vi "Start.vi"(1 "Engine":refnum<k7>, 2 "Context":refnum<k7>) -> (0 "Error Out":errorcluster)   [LabVIEW 2021, in "Seq Edit Quick Drop.lvlib"]
uses:
  Seq Edit Quick Drop.lvlib
  Command.ctl
  Data.ctl
  Register Item.ctl
  Message.ctl
  Event Response.ctl
  Connection Type.ctl
  Combine Key with Modifiers.vi
  Get Modifier from Key Event.vi
  Get Modifier.vi
  Scan Codes Mapping.vi
  <vilib>/Utility/error.llb/Trim Whitespace.vi
  Settings.vi
  <vilib>/Utility/SystemLogging/NI_SystemLogging.lvlib
  Resources/Tool Menu Utility.lvlibp/Tools/Tools.lvclass
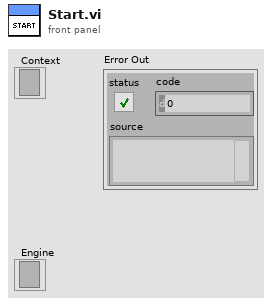
[diagram p1: front panel]
types:
  T1 = typedef "Seq Edit Quick Drop.lvlib/Message.ctl" = cluster{"cmd":T2, "data":variant}
  T2 = typedef "Seq Edit Quick Drop.lvlib/Command.ctl" = enum16{"Init", "Get Application Manager", "Shortcut Activated", "Display Tools", "Tool Selected", "Timeout", "Error", "Close"}
  T3 = typedef "Seq Edit Quick Drop.lvlib/Data.ctl" = cluster{"Engine":refnum<k7>, "Context":refnum<k7>, "Application Manager":refnum<k7>, "Register":map{string, T4}, "All Default Shortcuts":string[], "All Possible Shortcuts":string[], "Keys Mapping":map{string, string}, "Status Monitor":cluster{"Sequence Context":refnum<k7>, "Execution":refnum<k7>, "Termination Monitor":refnum<k7>}}
  T4 = typedef "Seq Edit Quick Drop.lvlib/Register Item.ctl" = cluster{"Id":i32, "Path":string, "Events":refnum<k27>[]}
  T5 = typedef "Seq Edit Quick Drop.lvlib/Event Response.ctl" = cluster{"Connection Type":T6, "ID":i32}
  T6 = typedef "Seq Edit Quick Drop.lvlib/Connection Type.ctl" = enum16{"SequenceView", "SequenceList", "VariablesView"}
  T7 = typedef "TestStand - Status Monitor.ctl" = cluster{"Sequence Context":refnum<k7>, "Execution":refnum<k7>, "Termination Monitor":refnum<k7>}
  T8 = cluster{"All Default Shortcuts":string[], "All Possible Shortcuts":string[], "Keys Mapping":map{string, string}}
  T9 = cluster{"Sequence Context":refnum<k7>, "Execution":refnum<k7>, "Termination Monitor":refnum<k7>}
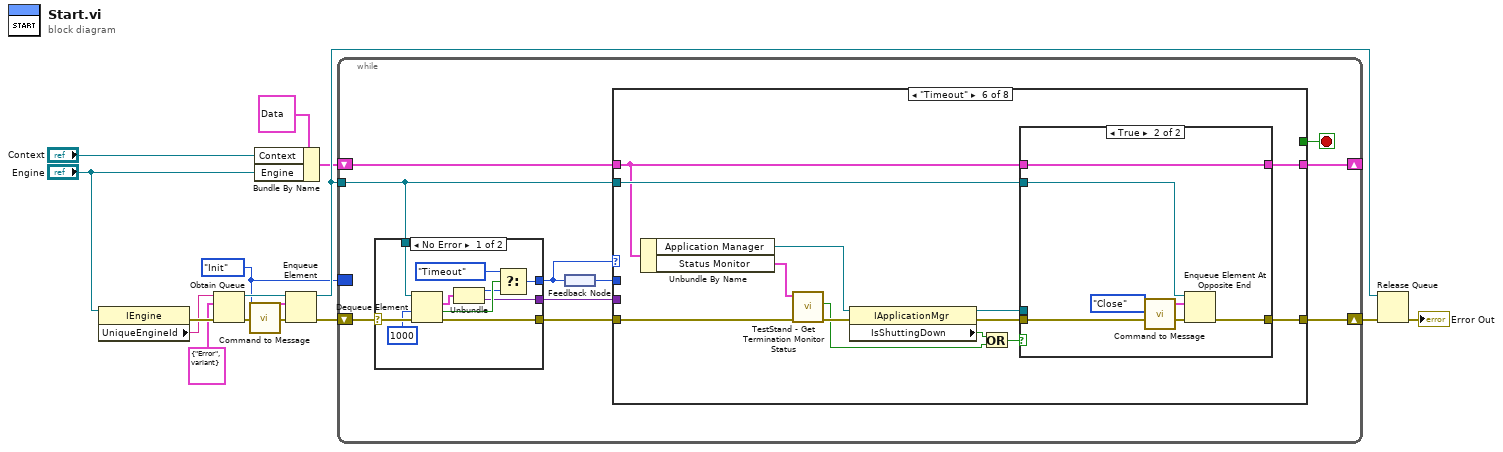
[diagram p0: block diagram]
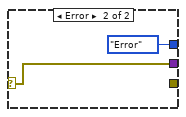
[diagram p2: hidden frame]
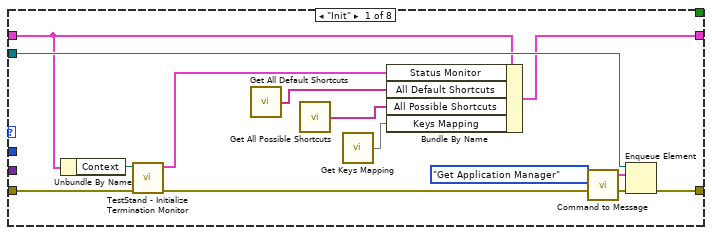
[diagram p3: hidden frame]
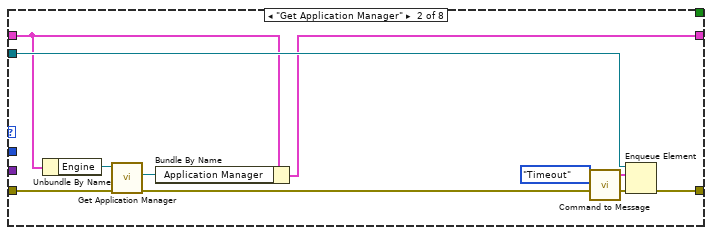
[diagram p4: hidden frame]
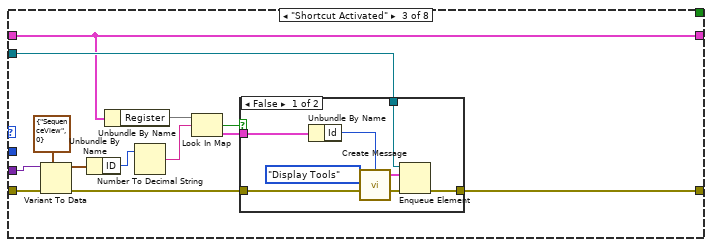
[diagram p5: hidden frame]
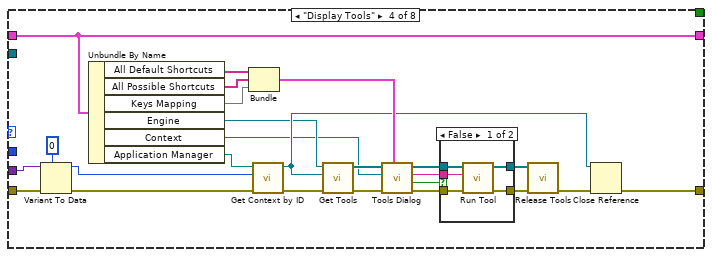
[diagram p7: hidden frame]
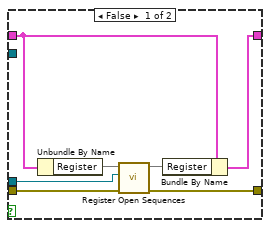
[diagram p10: hidden frame]
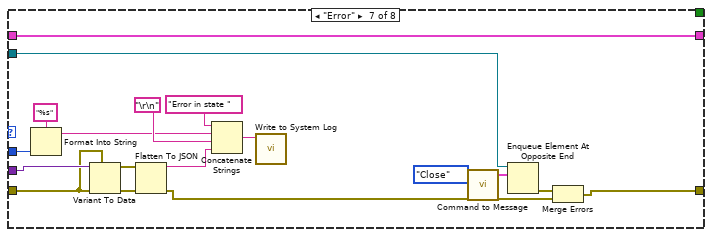
[diagram p11: hidden frame]
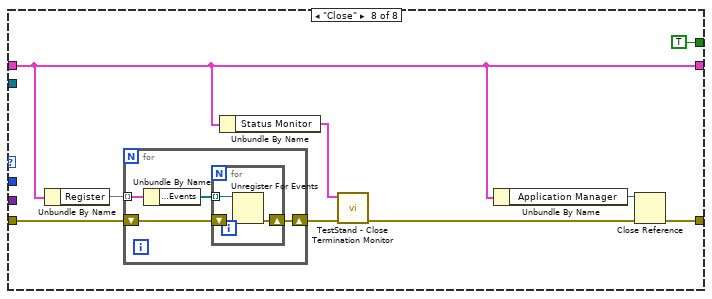
[diagram p12: hidden frame]
diagram:
  w5 = Command."Init" ("cmd")
  n1 = property class="IEngine"(reference="Engine") -> (error out=w14:errorcluster, "UniqueEngineId"=w1:string)  [unwired: 1 in, 1 out]
  n2 = Obtain Queue(name (unnamed)=w1, element data type=T1 {"cmd"=enum."Error", "data"=variant} ("cmd"), error in (no error)=w14) -> (queue out=w8:refnum<queue>, error out=w7:errorcluster)  [unwired: 2 in, 1 out]
  n3 = call "Command to Message.vi"("cmd"=w5) -> ("msg"=w4:T1)  [unwired: 4 in]
  n4 = Bundle By Name(cluster=T3 {"Engine"=refnum, "Context"=refnum, "Application Manager"=refnum, "Register"={}, "All Default Shortcuts"=[], "All Possible Shortcuts"=[], "Keys Mapping"={}, "Status Monitor"={"Sequence Context"=refnum, "Execution"=refnum, "Termination Monitor"=refnum}} ("Data"), "Context"="Context", "Engine"="Engine") -> (w11:T3)
  n5 = Enqueue Element(queue=w8, element=w4, error in (no error)=w7) -> (queue out=w15:refnum<queue>, error out=w6:errorcluster)  [unwired: 1 in, 1 out]
  n6 = while {
    border: w5 -> [_]
    shift-right: [w20] -> w13
    shift-left: w6 -> [w24]
    shift-right: [w17] -> _
    shift-left: w11 -> [w18]
    tunnel: w15 -> [w16]
    stop <- w19 stop-if-true
    n7 = case shown="No Error" w24 {
      selector: w24 -> [w35 w36]
      tunnel: [w32 Command."Error" ("cmd")] -> w21
      tunnel: [w34 _] -> w23
      tunnel: [w26 w36] -> w22
      tunnel: w16 -> [w29 _]
      frame No Error {
        n8 = Dequeue Element(queue=w29, timeout in ms (-1)=1000, error in (no error)=w35) -> (element=w28:T1, timed out?=w33:bool, error out=w34:errorcluster)  [unwired: 1 out]
        n9 = Unbundle(w28) -> ("cmd"=w27:T2, "data"=w26:variant)
        n10 = Select(t=Command."Timeout", s=w33, f=w27) -> (s? t:f=w32:T2)
      }
      frame Error {
      }
    }
    n11 = feedback #1() -> (w25:T2)
    n12 = feedback-in #1(w21) -> ()
    n13 = case shown="\"Timeout\"" w21 {
      tunnel: w25 -> [_ _ _ _ _ _ w147 _]
      tunnel: w23 -> [w50 w59 w72 w105 w115 w127 w150 w165]
      tunnel: w22 -> [_ _ w71 w103 _ _ w151 _]
      tunnel: [w49 w57 w61 w99 w115 w124 w143 w168] -> w20
      tunnel: [_ _ _ _ _ _ _ TRUE] -> w19
      tunnel: w18 -> [w40 w56 w67 w100 w114 w120 w158 w161]
      tunnel: [w42 w54 w67 w100 w114 w121 w158 w161] -> w17
      tunnel: w16 -> [w48 w60 w73 _ _ w128 w157 _]
      frame "Init" {
        n14 = Unbundle By Name(w40) -> ("Context"=w39:refnum<k7>)
        n15 = call <vilib>:"TestStand - Initialize Termination Monitor.vi"("error in (no error)"=w50, "Sequence Context In"=w39) -> ("error out"=w41:errorcluster, "Status Monitor Out"=w38:T7)  [unwired: 8 in]
        n16 = call "Get All Default Shortcuts.vi"() -> ("All Default Shortcuts"=w45:string[])
        n17 = call "Get All Possible Shortcuts.vi"() -> ("All Possible Shortcuts"=w44:string[])
        n18 = call "Get Keys Mapping.vi"() -> ("Keys Mapping"=w43:map{string, string})
        n19 = Bundle By Name(cluster=w40, "Status Monitor"=w38, "All Default Shortcuts"=w45, "All Possible Shortcuts"=w44, "Keys Mapping"=w43) -> (w42:T3)
        n20 = call "Command to Message.vi"("cmd"=Command."Get Application Manager") -> ("msg"=w47:T1)  [unwired: 4 in]
        n21 = Enqueue Element(queue=w48, element=w47, error in (no error)=w41) -> (error out=w49:errorcluster)  [unwired: 1 in, 2 out]
      }
      frame "Get Application Manager" {
        n22 = Unbundle By Name(w56) -> ("Engine"=w55:refnum<k7>)
        n23 = call "Get Application Manager.vi"("Error In"=w59, "Engine In"=w55) -> ("Error Out"=w58:errorcluster, "Application Manager"=w53:refnum<k7>)  [unwired: 7 in, 1 out]
        n24 = Bundle By Name(cluster=w56, "Application Manager"=w53) -> (w54:T3)
        n25 = call "Command to Message.vi"("cmd"=Command."Timeout") -> ("msg"=w51:T1)  [unwired: 4 in]
        n26 = Enqueue Element(queue=w60, element=w51, error in (no error)=w58) -> (error out=w57:errorcluster)  [unwired: 1 in, 2 out]
      }
      frame "Shortcut Activated" {
        n27 = Variant To Data(error in=w72, type=T5 {"Connection Type"=enum."SequenceView", "ID"=0} ("Event Response"), Variant=w71) -> (data=w69:T5, error out=w62:errorcluster)
        n28 = Unbundle By Name(w69) -> ("ID"=w68:i32)
        n29 = Unbundle By Name(w67) -> ("Register"=w66:map{string, T4})
        n30 = Number To Decimal String(number=w68) -> (decimal integer string=w65:string)  [unwired: 1 in]
        n31 = Look In Map(map=w66, key=w65) -> (key not found?=w63:bool, value=w64:T4)  [unwired: 1 in]
        n32 = case shown="False" w63 {
          tunnel: w64 -> [w80 _]
          tunnel: w62 -> [w79 w81]
          tunnel: [w78 w81] -> w61
          tunnel: w73 -> [w77 _]
          frame False {
            n33 = Unbundle By Name(w80) -> ("Id"=w75:i32)
            n34 = call "Create Message.vi"("cmd"=Command."Display Tools", "data"=w75) -> ("msg"=w76:T1)  [unwired: 2 in]
            n35 = Enqueue Element(queue=w77, element=w76, error in (no error)=w79) -> (error out=w78:errorcluster)  [unwired: 1 in, 2 out]
          }
          frame True {
          }
        }
      }
      frame "Display Tools" {
        n36 = Variant To Data(error in=w105, type=0, Variant=w103) -> (data=w101:i32, error out=w104:errorcluster)
        n37 = Unbundle By Name(w100) -> ("All Default Shortcuts"=w86:string[], "All Possible Shortcuts"=w85:string[], "Keys Mapping"=w84:map{string, string}, "Engine"=w93:refnum<k7>, "Context"=w82:refnum<k7>, "Application Manager"=w83:refnum<k7>)
        n38 = Bundle("All Default Shortcuts"=w86, "All Possible Shortcuts"=w85, "Keys Mapping"=w84) -> (w106:T8)  [unwired: 1 in]
        n39 = call "Get Context by ID.vi"("Error In"=w104, "Sequence ID"=w101, "Application Manager"=w83) -> ("Error Out"=w96:errorcluster, "Sequence Context"=w94:refnum<k7>)  [unwired: 7 in]
        n40 = call "Get Tools.vi"("Error In"=w96, "Context"=w94, "Engine"=w93) -> ("Error Out"=w95:errorcluster, "Tools"=w92:refnum<class "Tools.lvclass">[])  [unwired: 7 in]
        n41 = call "Tools Dialog.vi"("Settings"=w106, "Error In"=w95, "Context"=w82, "Tools In"=w92) -> ("Error Out"=w98:errorcluster, "Canceled?"=w88:bool, "ID"=w90:string, "Tools Out"=w89:refnum<class "Tools.lvclass">[])  [unwired: 4 in]
        n42 = case shown="False" w88 {
          tunnel: w98 -> [w111 w113]
          tunnel: [w110 w113] -> w97
          tunnel: w90 -> [w109 _]
          tunnel: w89 -> [w108 w112]
          tunnel: [w107 w112] -> w87
          frame False {
            n43 = call "Run Tool.vi"("Error In"=w111, "ID"=w109, "Tools In"=w108) -> ("Error Out"=w110:errorcluster, "Tools Out"=w107:refnum<class "Tools.lvclass">[])  [unwired: 7 in]
          }
          frame True {
          }
        }
        n44 = call "Release Tools.vi"("Error In"=w97, "Tools"=w87) -> ("Error Out"=w91:errorcluster)  [unwired: 9 in]
        n45 = Close Reference(reference=w94, error in (no error)=w91) -> (error out=w99:errorcluster)
      }
      frame "Tool Selected" {
        # "Placeholder case for executing super quick shorcuts"
        # "#TODO"
      }
      frame "Timeout" {
        n46 = Unbundle By Name(w120) -> ("Application Manager"=w123:refnum<k7>, "Status Monitor"=w118:T9)
        n47 = call <vilib>:"TestStand - Get Termination Monitor Status.vi"("error in (no error)"=w127, "Status Monitor In"=w118) -> ("error out"=w119:errorcluster, "Terminating or Aborting"=w116:bool)  [unwired: 7 in, 1 out]
        n48 = property class="IApplicationMgr"(reference=w123, error in=w119) -> (reference out=w122:refnum<k7>, error out=w125:errorcluster, "IsShuttingDown"=w126:bool)
        n49 = Or(x=w126, y=w116) -> (x .or. y?=w117:bool)
        n50 = case shown="True" w117 {
          tunnel: w125 -> [w135 w141]
          tunnel: [w134 w140] -> w124
          tunnel: w128 -> [_ w139]
          tunnel: w122 -> [w133 _]
          tunnel: w120 -> [w131 w136]
          tunnel: [w129 w136] -> w121
          frame False {
            n51 = Unbundle By Name(w131) -> ("Register"=w132:map{string, T4})
            n52 = call "Register Open Sequences.vi"("Error In"=w135, "Application Manager In"=w133, "Register In"=w132) -> ("Error Out"=w134:errorcluster, "Register Out"=w130:map{string, T4})  [unwired: 7 in]
            n53 = Bundle By Name(cluster=w131, "Register"=w130) -> (w129:T3)
          }
          frame True {
            n54 = call "Command to Message.vi"("cmd"=Command."Close") -> ("msg"=w137:T1)  [unwired: 4 in]
            n55 = Enqueue Element At Opposite End(queue=w139, element=w137, error in (no error)=w141) -> (error out=w140:errorcluster)  [unwired: 1 in, 2 out]
          }
        }
      }
      frame "Error" {
        n56 = Format Into String(format string="%s", w147) -> (resulting string=w146:string)  [unwired: 2 in, 1 out]
        n57 = Variant To Data(error in=w150, type=w150, Variant=w151) -> (data=w149:errorcluster, error out=w148:errorcluster)
        n58 = Flatten To JSON(anything=w149, error in (no error)=w148) -> (JSON string=w145:string, 11:w142:errorcluster)  [unwired: 1 in]
        n59 = Concatenate Strings("Error in state " ("string"), w146, "\r\n", w145) -> (w153:string)
        n60 = call <vilib>:"Write to System Log.vi"("message"=w153) -> ()  [unwired: 10 in, 1 out]
        n61 = call "Command to Message.vi"("cmd"=Command."Close") -> ("msg"=w155:T1)  [unwired: 4 in]
        n62 = Enqueue Element At Opposite End(queue=w157, element=w155) -> (error out=w159:errorcluster)  [unwired: 2 in, 2 out]
        n63 = Merge Errors(w159, w142) -> (w143:errorcluster)
      }
      frame "Close" {
        n64 = Unbundle By Name(w161) -> ("Register"=w164:map{string, T4})
        n65 = for {
          shift-right: [w172] -> w163
          shift-left: w165 -> [w171]
          tunnel: w164 -> [w170] mode=indexing
          n66 = Unbundle By Name(w170) -> ("Register Item.Events"=w169:refnum<k27>[])
          n67 = for {
            tunnel: w169 -> [w173] mode=indexing
            shift-right: [w175] -> w172
            shift-left: w171 -> [w174]
            n68 = Unregister For Events(event registration refnum=w173, error in=w174) -> (error out=w175:errorcluster)
          }
        }
        n69 = Unbundle By Name(w161) -> ("Status Monitor"=w160:T9)
        n70 = call <vilib>:"TestStand - Close Termination Monitor.vi"("error in (no error)"=w163, "Status Monitor In"=w160) -> ("error out"=w162:errorcluster)  [unwired: 9 in]
        n71 = Unbundle By Name(w161) -> ("Application Manager"=w167:refnum<k7>)
        n72 = Close Reference(reference=w167, error in (no error)=w162) -> (error out=w168:errorcluster)
      }
    }
  }
  n73 = Release Queue(queue=w15, error in (no error)=w13) -> (error out=→"Error Out":errorcluster)  [unwired: 1 in, 2 out]
